vi "test - Convert config array - null.vi"(8 "error in (no error)":errorcluster, 11 "TestCase in":refnum<class "Create New Assert Tester.lvclass">) -> (0 "error out":errorcluster, 3 "TestCase out":refnum<class "Create New Assert Tester.lvclass">)   [LabVIEW 2018, in "Create New Assert Tester.lvclass"]
uses:
  Create New Assert Tester.lvclass
  Plugins/Utility/Assert Build Configuration.ctl
  Core/Assert API Components/Failure Actions.ctl
  <vilib>/Utility/Data Type/Type Definitions/Data Type.ctl
  Plugins/Utility/Assert Scripting Configuration.ctl
  <vilib>/addons/_JKI Toolkits/VI Tester/TestCase.llb/TestCase.lvclass
  <vilib>/Utility/Data Type/NI_Data Type.lvlib
  Core/Assert API Components/Assert API Components.lvlib
  Plugins/Utility/Convert to scripting configuration.vi
  C:/Program Files (x86)/National Instruments/LabVIEW 2018/vi.lib/addons/_JKI Toolkits/VI Tester/TestCase.llb/TestCase.lvclass
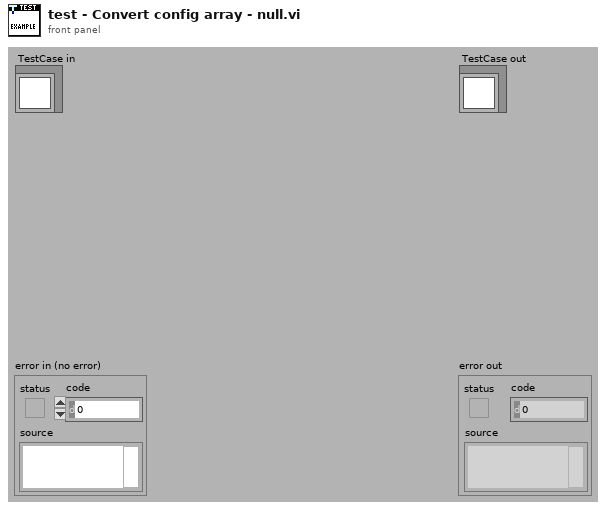
[diagram p1: front panel]
types:
  T1 = typedef "Assert Build Configuration.ctl" = cluster{"Assert Name":string, "Operation":string, "Comparison Value 1":string, "Comparison Value 2":string, "Comment":string, "Default Failure Action":T2, "Description":string, "Operation Display":string, "Active":bool, "Data Type":T3}
  T2 = typedef "Assert API Components.lvlib/Failure Actions.ctl" = enum16{"Display Only", "Log To File", "Pause Execution", "Abort Execution"}
  T3 = typedef "NI_Data Type.lvlib/Data Type.ctl" = enum8{"Invalid Type", "Void", "I8", "I16", "I32", "I64", "U8", "U16", "U32", "U64", "Single Float", "Double Float", "Extended Float", "Single Complex", "Double Complex", "Extended Complex", "Enum U8", "Enum U16", "Enum U32", "Enum U64", "Single Float With Unit", "Double Float With Unit", "Extended Float With Unit", "Single Complex with Unit", "Double Complex with Unit", "Extended Complex with Unit", "Boolean", "String", "Path", "Picture", "Tag", "Array", "Cluster", "Variant", "LV Variant", "Waveform", "Timestamp", "Digital Waveform", "Digital Data", "ExpressData", "Refnum", "External Data", "VI", "Poly VI", "LabVIEW Class Instance", "Fixed Point"}
  T4 = typedef "Assert Scripting Configuration.ctl" = cluster{"Assert Name":string, "Comment":string, "Numeric Operation":string, "Type":T3, "String Operation":string, "DBL Comparison Value 1":dbl, "DBL Comparison Value 2":dbl, "I32 Comparison Value 1":i32, "I32 Comparison Value 2":i32, "Creator":string, "Creation Timestamp":timestamp, "String Comparison Value":string, "Description":string, "Default Failure Action":enum16{"Display Only", "Log To File", "Pause Execution", "Abort Execution"}, "Boolean Comparison Value":bool, "I8 Comparison Value 1":i8, "I8 Comparison Value 2":i8, "I16 Comparison Value 1":i16, "I16 Comparison Value 2":i16, "I64 Comparison Value 1":i64, "I64 Comparison Value 2":i64, "U8 Comparison Value 1":u8, "U8 Comparison Value 2":u8, "U16 Comparison Value 1":u16, "U16 Comparison Value 2":u16, "U32 Comparison Value 1":u32, "U32 Comparison Value 2":u32, "U64 Comparison Value 1":u64, "U64 Comparison Value 2":u64, "EXT Comparison Value 1":ext, "EXT Comparison Value 2":ext, "SGL Comparison Value 1":sgl, "SGL Comparison Value 2":sgl, "Float Digits of Precision":u8}
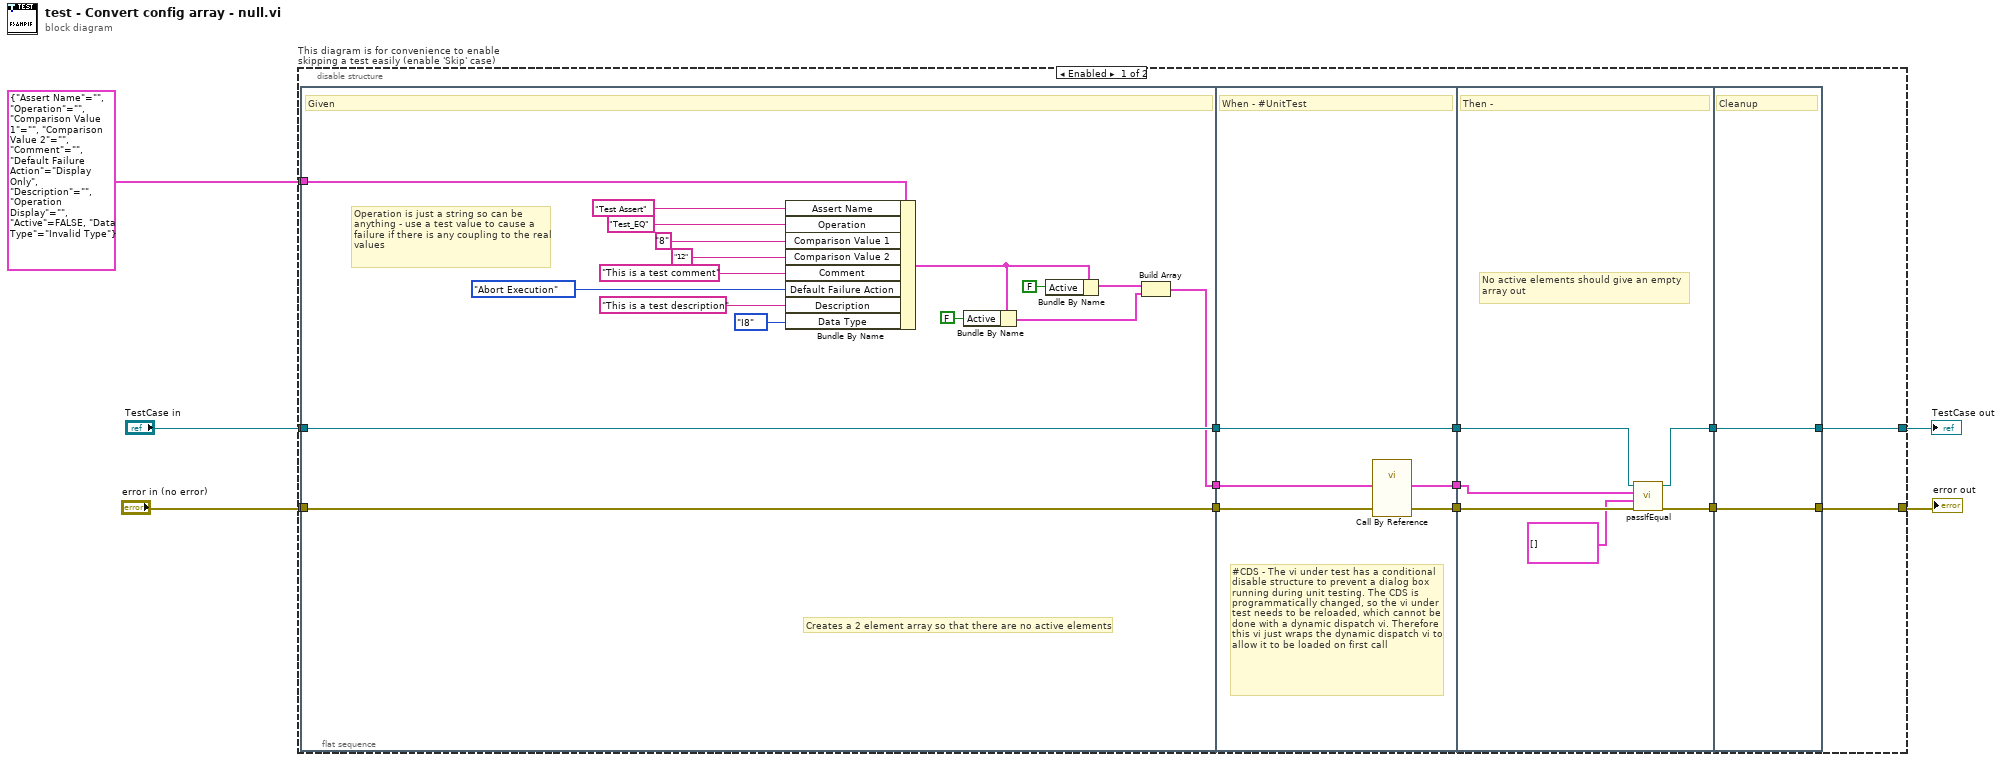
[diagram p0: block diagram]
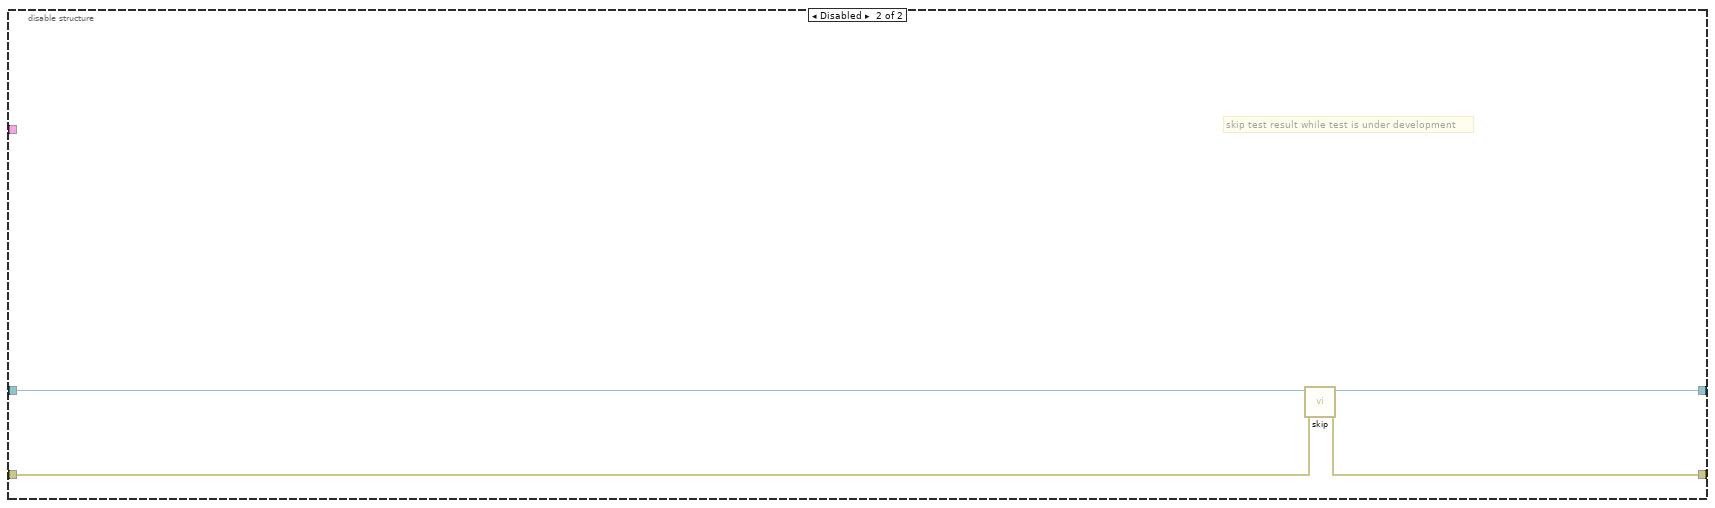
[diagram p2: hidden frame]
diagram:
  n1 = disable-structure "This diagram is for convenience to enable skipping a test easily (enable 'Skip' case)" shown="Enabled" {
    disable-tunnel: "TestCase in" -> [w12 w52]
    disable-tunnel: [w9 w50] -> w2
    disable-tunnel: [w10 w51] -> w4
    disable-tunnel: "error in (no error)" -> [w11 w49]
    disable-tunnel: T1 {"Assert Name"="", "Operation"="", "Comparison Value 1"="", "Comparison Value 2"="", "Comment"="", "Default Failure Action"=enum."Display Only", "Description"="", "Operation Display"="", "Active"=FALSE, "Data Type"=enum."Invalid Type"} ("Assert Build Configuration") -> [w7 _]
    frame Enabled {
      n2 = flat-sequence {
        tunnel: w11 -> [w34]
        tunnel: w12 -> [w35]
        tunnel: [w35] -> w18
        tunnel: [w34] -> w17
        tunnel: w7 -> [w33]
        tunnel: [w24] -> w6
        tunnel: [w40] -> w16
        tunnel: [w38] -> w15
        tunnel: w18 -> [w40]
        tunnel: w17 -> [w39]
        tunnel: [w37] -> w8
        tunnel: w6 -> [w36]
        tunnel: [w42] -> w14
        tunnel: [w43] -> w13
        tunnel: w16 -> [w44]
        tunnel: w15 -> [w46]
        tunnel: w8 -> [w45]
        tunnel: [w47] -> w10
        tunnel: [w48] -> w9
        tunnel: w14 -> [w48]
        tunnel: w13 -> [w47]
        frame #0 {
          # "Creates a 2 element array so that there are no active elements"
          # "Operation is just a string so can be anything - use a test value to cause a failure if there is any coupling to the real values"
          # "Given"
          n3 = Bundle By Name(cluster=w33, "Assert Name"="Test Assert", "Operation"="Test_EQ", "Comparison Value 1"="8" ("Comparison Value (Low)"), "Comparison Value 2"="12" ("Comparison Value (High)"), "Comment"="This is a test comment", "Default Failure Action"=Failure_Actions."Abort Execution", "Description"="This is a test description" ("Comment"), "Data Type"=Data_Type."I8") -> (w21:T1)
          n4 = Bundle By Name(cluster=w21, "Active"=FALSE) -> (w19:T1)
          n5 = Bundle By Name(cluster=w21, "Active"=FALSE) -> (w23:T1)
          n6 = Build Array(w23, w19) -> (w24:T1[])
        }
        frame #1 {
          # "#CDS - The vi under test has a conditional disable structure to prevent a dialog box running during unit testing. The CDS is programmatically changed, so the vi under test needs to be reloaded, which cannot be done with a dynamic dispatch vi. Therefore this vi just wraps the dynamic dispatch vi to allow it to be loaded on first call"
          # "When - #UnitTest"
          n7 = call-by-ref "?"("error in (no error)"=w39, "Multiple Assert Configuration"=w36) -> ("error out"=w38:errorcluster, "Array"=w37:T4[])  [unwired: 9 in, 3 out]
        }
        frame #2 {
          # "No active elements should give an empty array out"
          # "Then -"
          n8 = call-dynamic "passIfEqual.vi"("error in (no error)"=w46, "y"=T4[] [] ("Array"), "x"=w45, "TestCase in"=w44) -> ("error out"=w43:errorcluster, "TestCase out"=w42:refnum<class "Create New Assert Tester.lvclass">)  [unwired: 6 in]
        }
        frame #3 {
          # "Cleanup"
        }
      }
    }
    frame Disabled {
      # "skip test result while test is under development"
      n9 = call <vilib>:"skip.vi"("error in (no error)"=w49, "TestCase in"=w52) -> ("error out"=w51:errorcluster, "TestCase out"=w50:refnum<class "Create New Assert Tester.lvclass">)  [unwired: 8 in]
    }
  }
  "error out" <- w4
  "TestCase out" <- w2
